vi "Controller.vi"() -> ()   [LabVIEW 2018]
uses:
  <vilib>/Platform/TimedLoop/XDataNode/timing_clust.ctl
  <vilib>/Platform/TimedLoop/XDataNode/nitl_modes.ctl
  <vilib>/Platform/TimedLoop/XDataNode/wakeup.ctl
  <vilib>/Modbus/master/Create Master Instance (TCP).vi
  <vilib>/Modbus/slave/Create Slave Instance (TCP).vi
  <vilib>/Platform/TimedLoop/XDataNode/XDataNode.xnode
  <vilib>/Modbus/slave/Modbus Slave.lvclass
  <vilib>/Modbus/master/Modbus Master.lvclass
  <vilib>/Platform/TimedLoop/XDataNode/XDNodeRunTimeDep.lvlib
panel:
  out "BPCS-FJ":dbl
  out "BPCS-HMI-TX-ARRAY":dbl[](array[numeric])
  out "SIS-BPCS-RX-Array":bool[](array[boolean])
  out "BPCS-SIM-TX-ARRAY":dbl[](array[numeric])
  out "error out":errorcluster
  in  "stop":bool
  out "BPCS-10TY100":dbl format="%.2f"
  out "BPCS-10AY300":dbl
  out "BPCS-SIM-TX-ARRAY":dbl[](array[numeric])
  out "BPCS-10Y200":dbl format="%.2f"
  out "HMI-10HIC100":dbl
  out "HMI-10TIC100-SP":dbl
  out "HMI-10TIC100-KPID":dbl[](array[numeric])=[1.0, 0.01, 0.0]
  out "HMI-10HIC200":dbl
  out "HMI-10LIC200-SP":dbl
  out "HMI-10LIC200-KPID":dbl[](array[numeric])
  out "HMI-10HIC300":dbl
  out "HMI-10TIC100_MA":bool
  out "HMI-10LIC200_MA":bool
  out "SIS-10SDV501":bool
  out "SIS-10SDV500":bool
  out "SIS-10SDV502":bool
  out "BPCS-10LI200":dbl
  out "SIM-BPCS-RX-ARRAY":dbl[](array[numeric])
  out "BPCS-10TI100":dbl
  # "T0"
  # "CA0"
  # "TJ0"
  # "F"
  # "FJ"
  # "L"
  # "CA"
  # "T"
  # "TJ"
  # "F0"
  # "BPCS-10Y200"
  # "BPCS-10TY100"
  # "BPCS-10AY300"
  # "SIS-10SDV500"
  # "SIS-10SDV501"
  # "SIS-10SDV502"
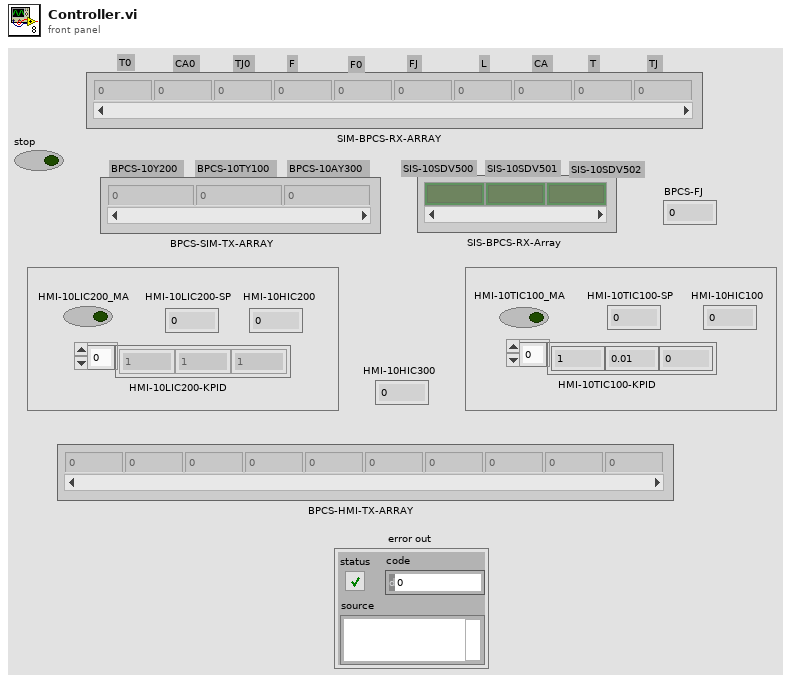
[diagram p1: front panel]
types:
  T1 = typedef "XDNodeRunTimeDep.lvlib/timing_clust.ctl" = cluster{"Expected End [f-1]":u64, "Actual End [f-1]":u64, "Finished Late? [f-1]":bool, "Expected End [i-1]":u64, "Actual End [i-1]":u64, "Finished Late? [i-1]":bool, "Expected Start [i]":u64, "Actual Start [i]":u64, "Expected Start [f]":u64, "Actual Start [f]":u64, "Source Name":string, "Structure Name":string, "Period":i64, "Deadline":i64, "Offset":i64, "Start":i64, "Priority":i32, "Timeout":i32, "Mode":T2, "Wakeup Reason":T3, "Error":errorcluster, "Source Type":string, "Secondary Source Type":string, "Global End Time":u64, "Global Start Time":u64, "Frame Duration":u64, "Iteration Duration":u64, "Assigned CPU":i32, "I/O Scan Engine Mode":u32}
  T2 = typedef "XDNodeRunTimeDep.lvlib/nitl_modes.ctl" = enum32{"No Change", "Process missed periods, maintain original phase", "Discard missed periods, maintain original phase", "Process missed periods, ignore original phase", "Discard missed periods, ignore original phase"}
  T3 = typedef "XDNodeRunTimeDep.lvlib/wakeup.ctl" = enum32{"Normal", "Aborted", "Asynchronous wakeup", "Timing source error", "Timed loop error", "Timeout"}
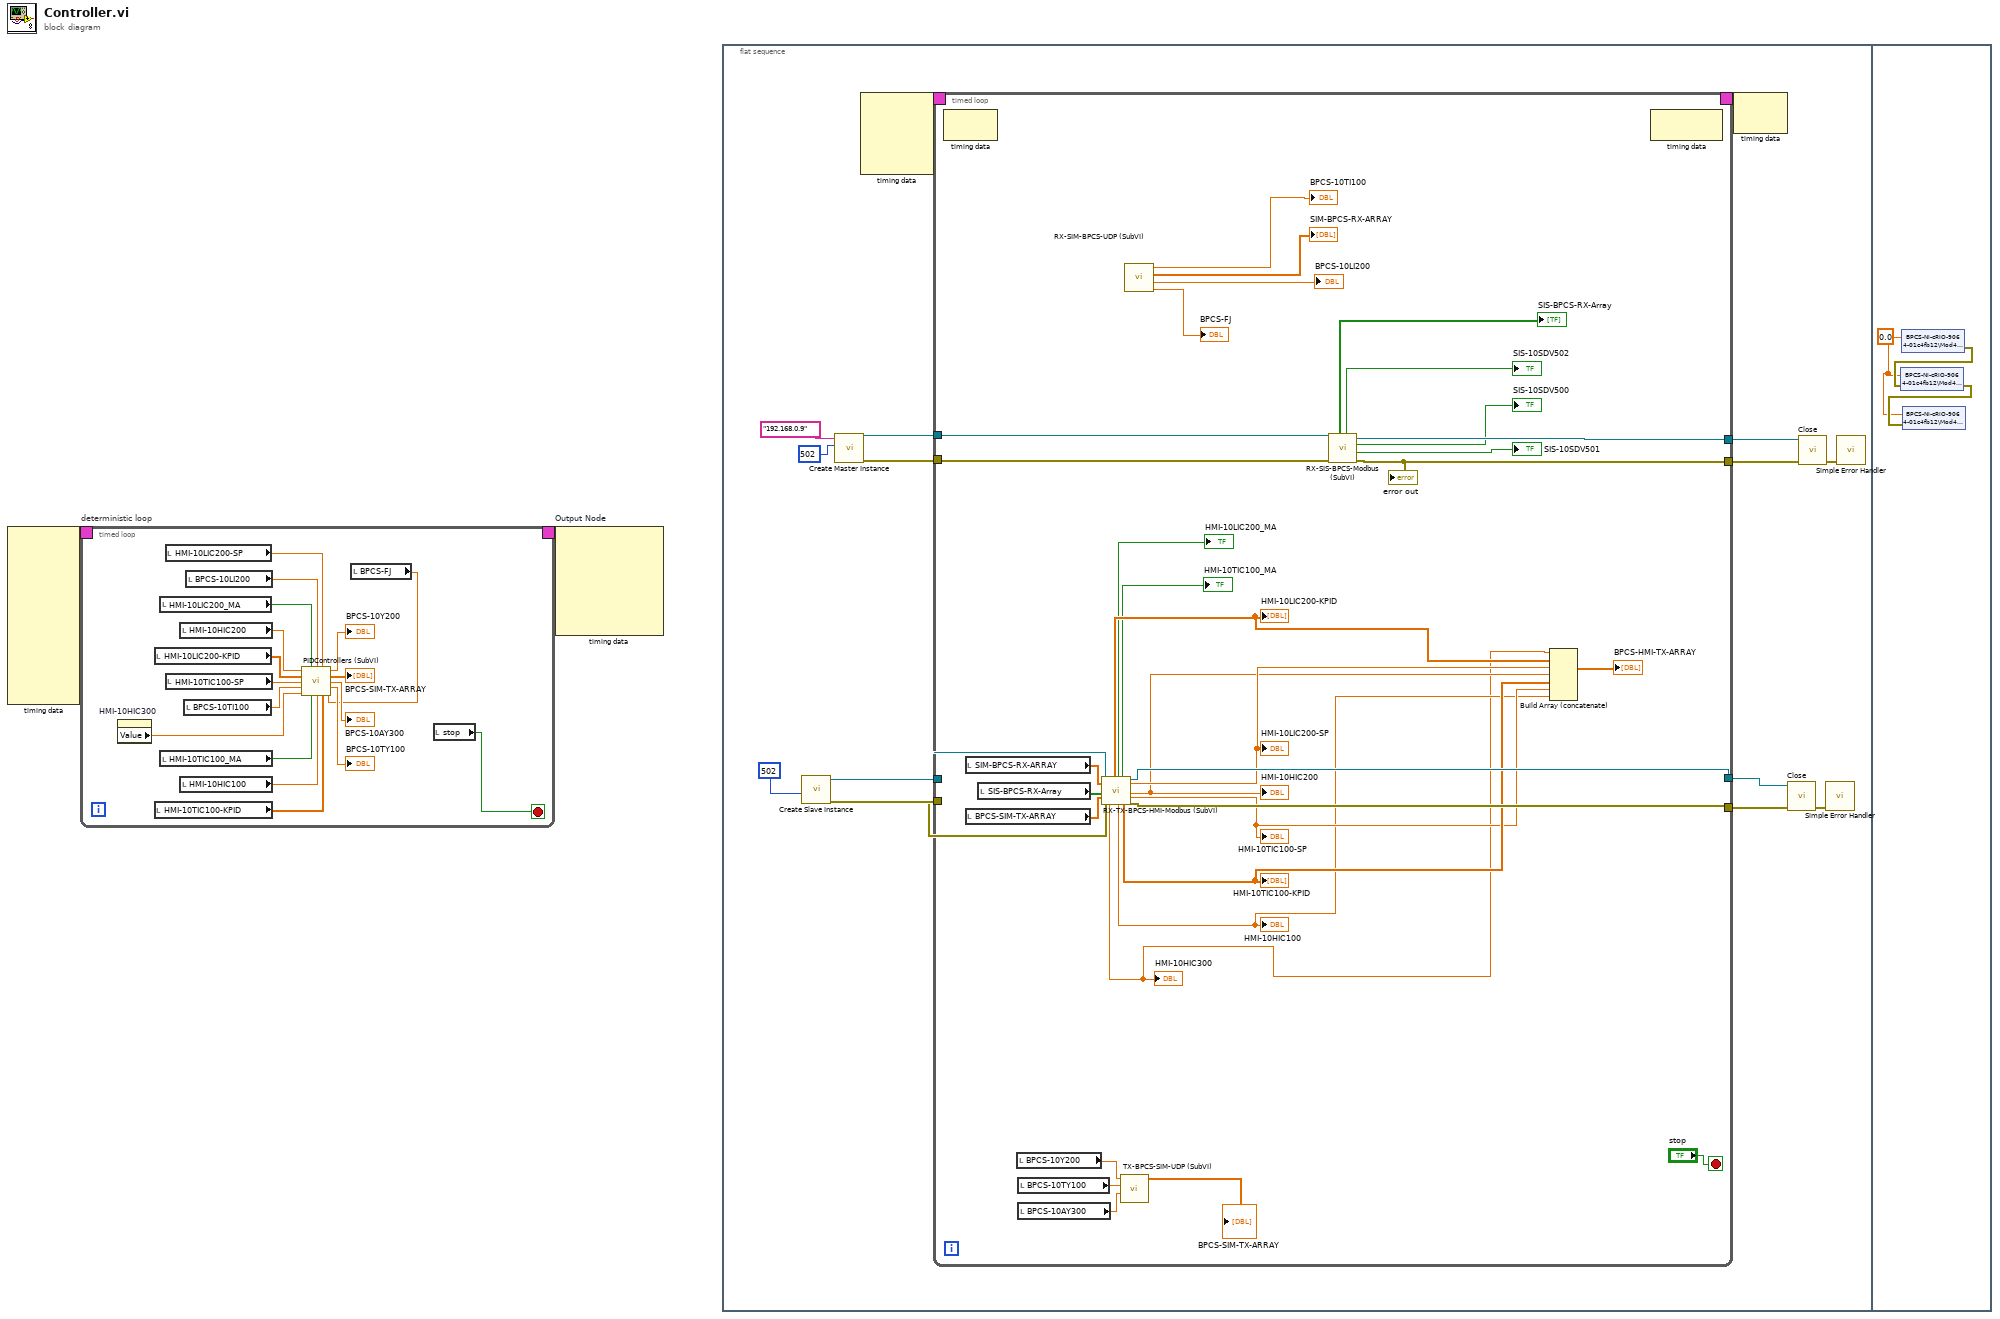
[diagram p0: block diagram]
diagram:
  n1 = node-c288 ("Input Node")() -> (w2:T1)  [unwired: 10 in]
  n2 = timed-loop "deterministic loop" {
    timing: w2 -> [_]
    timing-out: [_] -> w1
    stop <- w5 stop-if-true
    n3 = property on="HMI-10HIC300" class="DigNum (strict)"() -> ("Value"=w4:dbl)  [unwired: 2 in, 2 out]
    n4 = local read "HMI-10LIC200-KPID"() -> (w15:dbl[])
    n5 = local read "HMI-10TIC100-KPID"() -> (w10:dbl[])
    n6 = local read "HMI-10LIC200_MA"() -> (w17:bool)
    n7 = local read "HMI-10TIC100_MA"() -> (w12:bool)
    n8 = local read "HMI-10LIC200-SP"() -> (w19:dbl)
    n9 = local read "HMI-10TIC100-SP"() -> (w14:dbl)
    n10 = local read "HMI-10HIC200"() -> (w16:dbl)
    n11 = local read "HMI-10HIC100"() -> (w11:dbl)
    n12 = local read "BPCS-10TI100"() -> (w13:dbl)
    n13 = local read "BPCS-10LI200"() -> (w18:dbl)
    n14 = local read "BPCS-FJ"() -> (w3:dbl)
    n15 = call "PIDControllers (SubVI).vi"("HMI-10HIC200"=w16, "HMI-10LIC200_MA"=w17, "BPCS-10LI200"=w18, "HMI-10LIC200-SP"=w19, "HMI-10LIC200-KPID"=w15, "HMI-10TIC100-SP"=w14, "BPCS-10TI100"=w13, "HMI-10HIC300"=w4, "HMI-10TIC100_MA"=w12, "HMI-10HIC100"=w11, "HMI-10TIC100-KPID"=w10, "BPCS-FJ"=w3) -> ("BPCS-10Y200"=→"BPCS-10Y200":dbl, "BPCS-SIM-TX-ARRAY"=→"BPCS-SIM-TX-ARRAY":dbl[], "BPCS-10AY300"=→"BPCS-10AY300":dbl, "BPCS-10TY100"=→"BPCS-10TY100":dbl)
    n16 = local read "stop"() -> (w5:bool)
  }
  n17 = node-c288 "Output Node"(w1) -> ()  [unwired: 6 out]
  n18 = flat-sequence {
    frame #0 {
      n19 = call-poly <vilib>:"Create Slave Instance.vi"("port (502)"=u16 502) -> ("error out"=w32:errorcluster, "TCP slave instance"=w33:refnum<class "Modbus Slave.lvclass">)  [unwired: 9 in]
      n20 = call-poly <vilib>:"Create Master Instance.vi"("port (502)"=u16 502, "address"="192.168.0.9") -> ("error out"=w25:errorcluster, "TCP master instance"=w26:refnum<class "Modbus Master.lvclass">)  [unwired: 8 in]
      n21 = node-c288() -> (w24:T1)  [unwired: 4 in]
      n22 = timed-loop {
        tunnel: [w61] -> w35
        tunnel: [w60] -> w34
        tunnel: w33 -> [w68]
        tunnel: [w63] -> w30
        tunnel: w32 -> [w67]
        tunnel: [w62] -> w29
        tunnel: w26 -> [w59]
        tunnel: w25 -> [w58]
        timing: w24 -> [_]
        timing-out: [_] -> w23
        stop <- "stop" stop-if-true
        n23 = node-c288() -> ()  [unwired: 1 in, 1 out]
        n24 = local read "SIM-BPCS-RX-ARRAY"() -> (w66:dbl[])
        n25 = local read "BPCS-SIM-TX-ARRAY"() -> (w64:dbl[])
        n26 = local read "SIS-BPCS-RX-Array"() -> (w65:bool[])
        n27 = local read "BPCS-10Y200"() -> (w54:dbl)
        n28 = local read "BPCS-10TY100"() -> (w53:dbl)
        n29 = local read "BPCS-10AY300"() -> (w52:dbl)
        n30 = call "RX-TX-BPCS-HMI-Modbus (SubVI).vi"("Modbus Slave in"=w68, "SIM-BPCS-RX-ARRAY"=w66, "SIS-BPCS-RX-Array"=w65, "BPCS-SIM-TX-ARRAY"=w64, "error in (no error)"=w67) -> ("HMI-10HIC300"=w40:dbl, "HMI-10LIC200-KPID"=w47:dbl[], "HMI-10LIC200_MA"=→"HMI-10LIC200_MA":bool, "HMI-10HIC100"=w42:dbl, "HMI-10TIC100_MA"=→"HMI-10TIC100_MA":bool, "HMI-10TIC100-KPID"=w44:dbl[], "Modbus Slave out"=w63:refnum<class "Modbus Slave.lvclass">, "HMI-10LIC200-SP"=w46:dbl, "HMI-10HIC200"=w45:dbl, "HMI-10TIC100-SP"=w43:dbl, "error out"=w62:errorcluster)  [unwired: 4 in]
        "HMI-10LIC200-KPID" <- w47
        "HMI-10LIC200-SP" <- w46
        "HMI-10HIC200" <- w45
        "HMI-10TIC100-KPID" <- w44
        "HMI-10TIC100-SP" <- w43
        "HMI-10HIC100" <- w42
        "HMI-10HIC300" <- w40
        n31 = call "TX-BPCS-SIM-UDP (SubVI).vi"("BPCS-10AY300"=w52, "BPCS-10TY100"=w53, "BPCS-10Y200"=w54) -> ("BPCS-SIM-TX-ARRAY"=→"BPCS-SIM-TX-ARRAY":dbl[])  [unwired: 8 in]
        n32 = call "RX-SIM-BPCS-UDP (SubVI).vi"() -> ("BPCS-FJ"=→"BPCS-FJ":dbl, "BPCS-10LI200"=→"BPCS-10LI200":dbl, "SIM-BPCS-RX-ARRAY"=→"SIM-BPCS-RX-ARRAY":dbl[], "BPCS-10TI100"=→"BPCS-10TI100":dbl)  [unwired: 8 in]
        n33 = call "RX-SIS-BPCS-Modbus (SubVI).vi"("error in (no error)"=w58, "Modbus Master in"=w59) -> ("error out"=w60:errorcluster, "SIS-10SDV501"=→"SIS-10SDV501":bool, "SIS-10SDV500"=→"SIS-10SDV500":bool, "Modbus Master out"=w61:refnum<class "Modbus Master.lvclass">, "SIS-10SDV502"=→"SIS-10SDV502":bool, "SIS-BPCS-RX-Array"=→"SIS-BPCS-RX-Array":bool[])  [unwired: 4 in]
        "error out" <- w60
        n34 = Build Array (concatenate)(w40, w47, w46, w45, w44, w43, w42) -> (→"BPCS-HMI-TX-ARRAY":dbl[])
        n35 = node-c288() -> ()  [unwired: 1 in, 1 out]
      }
      n36 = node-c288(w23) -> ()  [unwired: 1 out]
      n37 = call-dynamic "Close.vi"("error in (no error)"=w29, "Modbus slave in"=w30) -> ("error out"=w31:errorcluster)  [unwired: 9 in]
      n38 = call-dynamic "Close.vi"("error in (no error)"=w34, "Modbus master in"=w35) -> ("error out"=w36:errorcluster)  [unwired: 9 in]
      n39 = call <vilib>:"Simple Error Handler.vi"("error in (no error)"=w31) -> ()  [unwired: 4 in, 5 out]
      n40 = call <vilib>:"Simple Error Handler.vi"("error in (no error)"=w36) -> ()  [unwired: 4 in, 5 out]
    }
    frame #1 {
      w75 = 0.0 ("AO0")
      n41 = shared-variable "BPCS-NI-cRIO-9064-01c4fb12\\Mod4\\AO0"(w75) -> (error out=w77:errorcluster)  [unwired: 1 in]
      n42 = shared-variable "BPCS-NI-cRIO-9064-01c4fb12\\Mod4\\AO1"(w75, error in=w77) -> (error out=w76:errorcluster)
      n43 = shared-variable "BPCS-NI-cRIO-9064-01c4fb12\\Mod4\\AO2"(w75, error in=w76) -> ()  [unwired: 1 out]
    }
  }
